vi "setUp.vi"(8 "error in (no error)":errorcluster, 11 "reference in":refnum<class "BM Enable.lvclass">) -> (0 "error out":errorcluster, 3 "reference out":refnum<class "BM Enable.lvclass">)   [LabVIEW 2016, in "BM Enable.lvclass"]
doc: "setUp runs prior to the test method during test execution. Use this method to initialize any object data required by your tests."
uses:
  BM Enable.lvclass
  <vilib>/addons/_JKI Toolkits/VI Tester/TestCase.llb/TestCase.lvclass
  1553 Board/1553 Board.lvclass
  D:/SVN/Products/SLSC/Multichannel 1553 Module/Software/Source Code/Driver (Windows)/Unit Tests/1553 Test/1553 Test.lvclass
  D:/Programs/National Instruments/LabVIEW 2016/vi.lib/addons/_JKI Toolkits/VI Tester/TestCase.llb/TestCase.lvclass
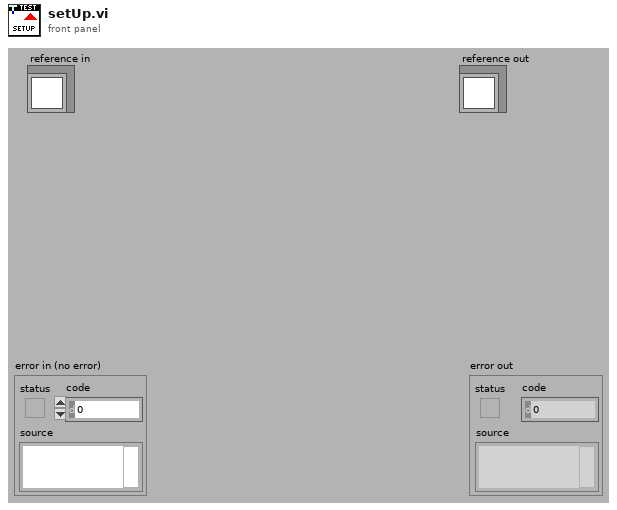
[diagram p1: front panel]
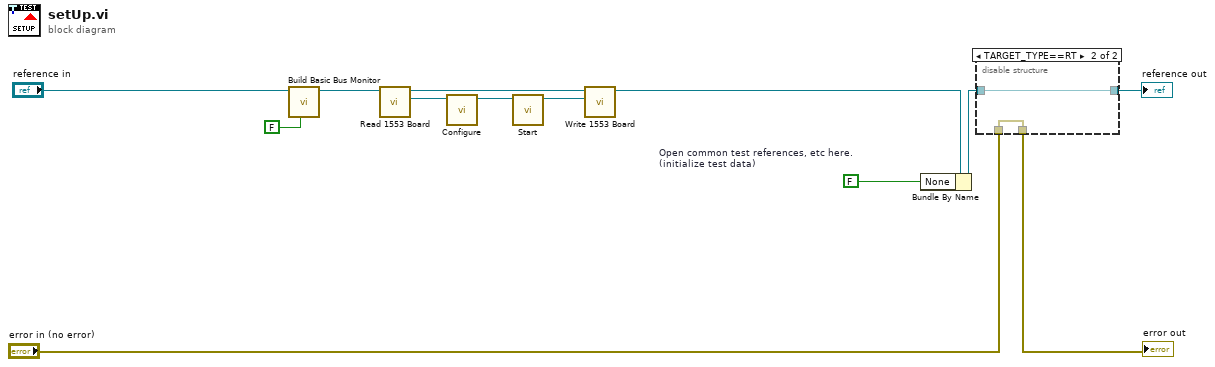
[diagram p0: block diagram]
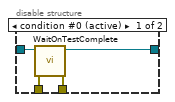
[diagram p2: hidden frame]
diagram:
  w9 = FALSE  # Open common test references, etc here. (initialize test data)
  n1 = call-dynamic "Build Basic Bus Monitor.vi"("48-bit Time Tag"=FALSE, "1553 Test in"="reference in") -> ("1553 Test out"=w4:refnum<class "BM Enable.lvclass">)  [unwired: 8 in, 1 out]
  n2 = call-dynamic "Read 1553 Board.vi"("1553 Test in"=w4) -> ("1553 Board"=w5:refnum<class "1553 Board.lvclass">, "1553 Test out"=w6:refnum<class "BM Enable.lvclass">)  [unwired: 8 in, 1 out]
  n3 = call-dynamic "Configure.vi"("1553 Board in"=w5) -> ("1553 Board out"=w2:refnum<class "1553 Board.lvclass">)  [unwired: 9 in, 1 out]
  n4 = call-dynamic "Start.vi"("1553 Board in"=w2) -> ("1553 Board out"=w1:refnum<class "1553 Board.lvclass">)  [unwired: 9 in, 1 out]
  n5 = call-dynamic "Write 1553 Board.vi"("1553 Board"=w1, "1553 Test in"=w6) -> ("1553 Test out"=w3:refnum<class "BM Enable.lvclass">)  [unwired: 8 in, 1 out]
  n6 = Bundle By Name(cluster=w3, "None"=w9) -> (w10:refnum<class "BM Enable.lvclass">)
  n7 = disable-structure shown="TARGET_TYPE==RT" {
    disable-tunnel: "error in (no error)" -> [w17 w18]
    disable-tunnel: [w16 w18] -> w12
    disable-tunnel: [w15 w19] -> w11
    disable-tunnel: w10 -> [w14 w19]
    frame condition #0 (active) {
      n8 = call <vilib>:"WaitOnTestComplete.vi"("error in (no error)"=w17, "TestCase in"=w14) -> ("error out"=w16:errorcluster, "TestCase out"=w15:refnum<class "BM Enable.lvclass">)  [unwired: 8 in]
    }
    frame condition #1 {
    }
  }
  "error out" <- w12
  "reference out" <- w11
